vi "复材超声C扫缺陷分析评定软件.vi"() -> ()   [LabVIEW 2018]
doc: "使用该模板构建用户界面事件处理设计模式。将模板应用于对话框及其它用户界面。用户也可创建并执行VI可按照与用户界面事件相同方式处理的用户定义事件。"
uses:
  <vilib>/Utility/NIReport.llb/Report Type.ctl
  <vilib>/addons/_office/_exclsub.llb/font.ctl
  <vilib>/addons/_office/word.llb/Word Easy Table (str).vi
  <vilib>/Utility/NIReport.llb/Append Image to Report (path wrap).vi
  <vilib>/Utility/NIReport.llb/NI_report.lvclass
  <vilib>/Utility/NIReport.llb/Append Report Text (str wrap).vi
  <vilib>/vision/NI_Vision_Development_Module.lvlib
  <vilib>/Utility/NIReport.llb/NI_ReportGenerationCore.lvlib
  <vilib>/addons/_office/NI_ReportGenerationToolkit.lvlib
panel:
  out "连接的字符串 2":string
  out "临界面积百分比值":dbl
  out "临界Z值":i32
  out "true":bool
  out "标注后的图片路径":path
  out "弥散类检测结果合并":string[][](table)
  out "分层类检测结果合并":string[][](table)
  out "反射图原始路径":path
  out "穿透图原始路径":path
  out "弥散类检测结果":string[][](table)
  out "分层类检测结果":string[][](table)
  out "部位信息":string[](array[string])=["", "34.500000", "32.500000", "1121", "34", "54.955926", "分层类", "不合格", ""]
  out "连接的字符串":string
  in  "完成标注":bool caption="定量分析"
  out "框数":dbl
  in  "Operation":enum16{"overlay rectangle"}(ring)
  out "ROI左上角坐标":cluster{i32, i32}
  out "自定义字体":T1={"Desired Font (Application)"=enum."Application Font", "[User-specified Font]"={"Font Name"="", "Size"=12, "Strikeout?"=FALSE, "Italic?"=FALSE, "Underline?"=FALSE, "Outline?"=FALSE, "Shadow?"=FALSE, "Bold?"=FALSE, "Rotation Angle"=0.0}, "Horizontal Alignment"=0, "Vertical Alignment"=0} {"Horizontal Alignment" items=["Left", "Center", "Right"]; "Vertical Alignment" items=["Bottom", "Top", "Baseline"]}
  out "标注图ROI2Mask":T2(plugin-control)
  out "透射图最大灰度值":sgl
  out "反射图最大灰度值":sgl
  out "反射图灰度表":u32[](graph)
  out "透射图灰度表":u32[](graph)
  out "总面积":i32
  out "框组":T3(array[cluster])
  out "质量等级":string
  in  "导入反射图":bool caption="导入图片"
  out "灰度阈值":dbl
  in  "stop":bool caption="停止"
  in  "导入穿透图":bool caption="导入图片"
  in  "图像预处理":bool
  in  "自定义色彩":bool
  in  "缺陷标注":bool caption="定量分析"
  in  "查看标注":bool caption="辅助定性分析"
  in  "生成评定结果":bool caption="生成原始记录"
  in  "?":enum32{"穿透图", "反射图"}(tab)
  out "穿透图":T2(plugin-control)
  out "反射图":T2(plugin-control)
  out "产品规格":cluster{"产品长度（周长）（mm）":dbl, "产品宽度（母线长）（mm）":dbl}
  out "图像分辨率":T4
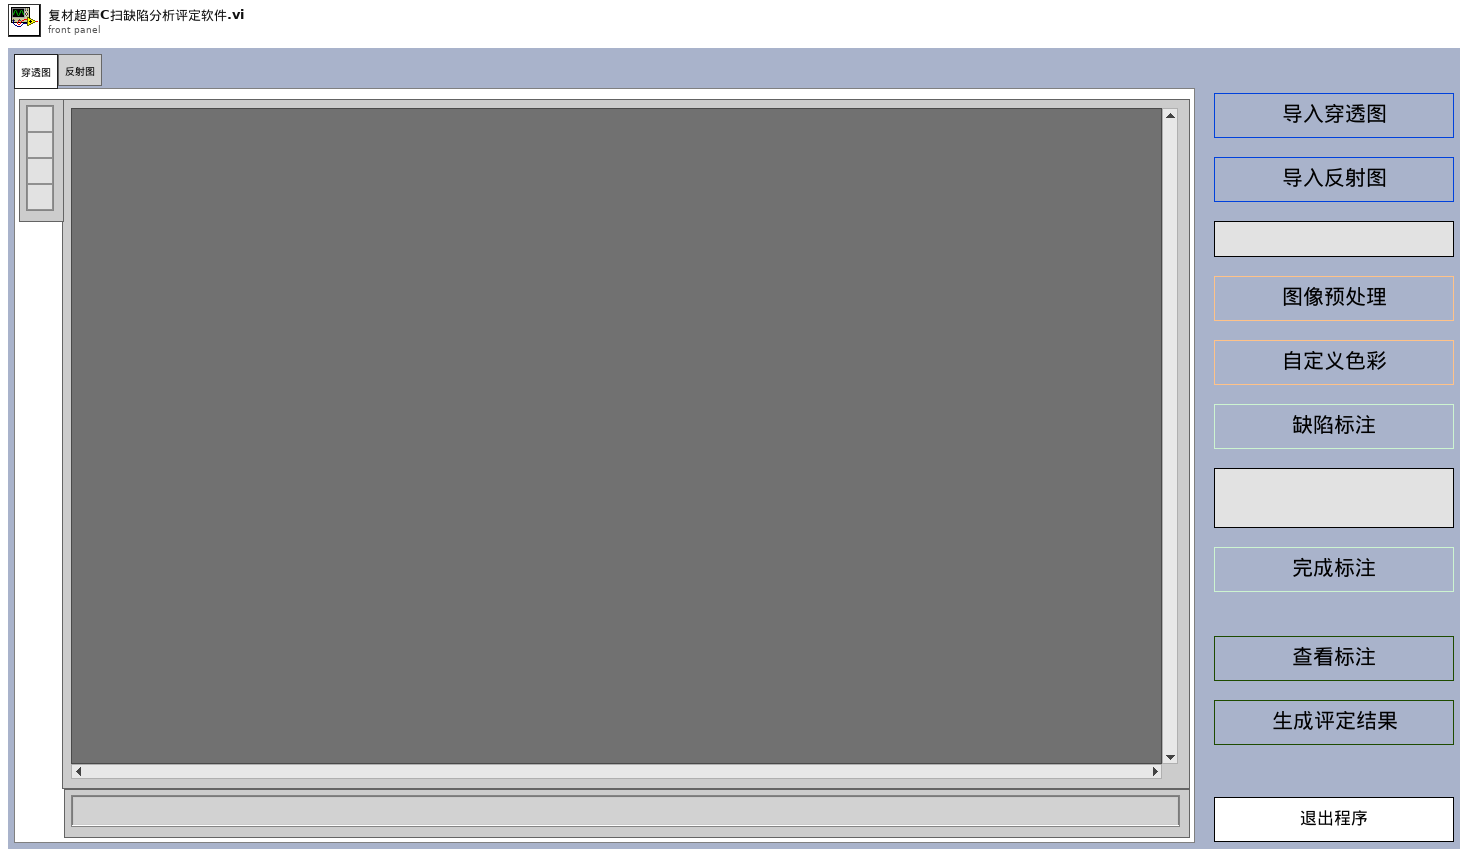
[diagram p1: front panel]
types:
  T1 = cluster{"Desired Font (Application)":enum16{"User-specified Font", "Application Font", "System Font", "Dialog Font"}, "[User-specified Font]":cluster{"Font Name":string, "Size":i16, "Strikeout?":bool, "Italic?":bool, "Underline?":bool, "Outline?":bool, "Shadow?":bool, "Bold?":bool, "Rotation Angle":dbl}, "Horizontal Alignment":i16, "Vertical Alignment":i16}
  T2 = typedef "IMAQ Image.ctl" = refnum<image>
  T3 = cluster{"Global Rectangle":i32[], "Contours":cluster{"Contour Type":u32, "ROI Type":u32, "Points":i32[]}[]}[]
  T4 = cluster{"图像X向分辨率（mm/像素）":dbl, "图像Y向分辨率（mm/像素）":dbl}
  T5 = cluster{"Zoom Tool":bool, "Selection Tool":bool, "Pan Tool":bool, "Point Tool":bool, "Line Tool":bool, "Rectangle Tool":bool, "Rotated Rectangle Tool":bool, "Polyline Tool":bool, "Polygon Tool":bool, "Freehand Tool":bool, "Closed Freehand Tool":bool, "Ellipse Tool":bool, "Annulus Tool":bool}
  T6 = enum32{"Invalid", "Standard", "Closed", "Hidden", "Minimized", "Maximized"}
  T7 = enum32{"Linear", "Log", "Exp", "Square", "Square root", "Power X", "Power 1/X"}
  T8 = enum32{"Gray", "Binary", "Gradient", "Rainbow", "Temperature"}
  T9 = cluster{"position (excel)":cluster{"row":i32, "column":i32}, "name (excel)":string, "bookmark (word)":string}
  T10 = typedef "NI_ReportGenerationToolkit.lvlib/font.ctl" = cluster{"font name":string, "font size":dbl, "bold":u16, "italic":u16, "underline":u16, "strike through":u16, "font color":u32}
  T11 = enum16{"maximized", "minimized", "normal", "no change"}
  T12 = typedef "NI_ReportGenerationCore.lvlib/Report Type.ctl" = enum16{"HTML", "Word", "Excel"}
  T13 = cluster{"position (Excel)":cluster{"row":i32, "column":i32}, "name (Excel)":string, "bookmark (Word)":string}
  T14 = typedef "Image Type" = u32
  T15 = cluster{"Red (or Hue) value":u8, "Green (or Sat) value":u8, "Blue (or Light or Val) value":u8}[]
  T16 = cluster{"histogram":u32[], "Minimal Value":sgl, "Maximal Value":sgl, "Starting Value":sgl, "Interval Width":sgl, "Mean Value":sgl, "Standard  Variation":sgl, "Area (pixels)":i32}
  T17 = cluster{"Global Rectangle":i32[], "Contours":cluster{"Contour Type":u32, "ROI Type":u32, "Points":i32[]}[]}
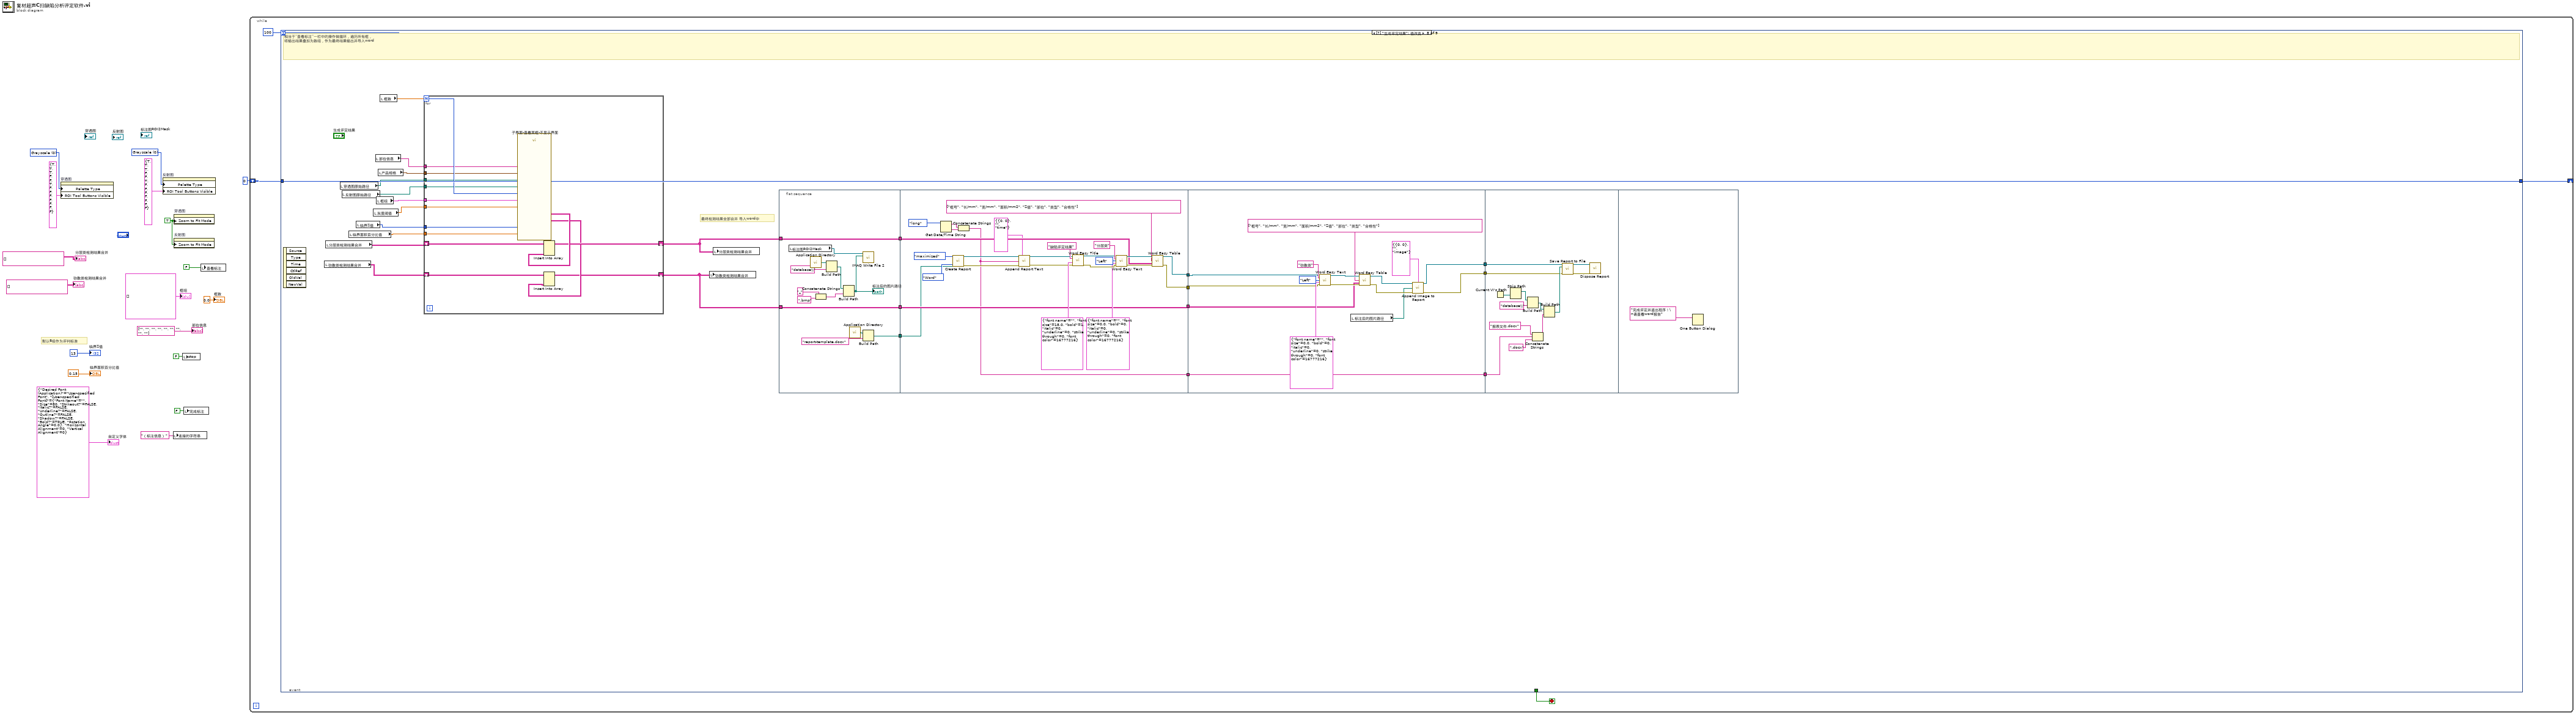
[diagram p0: block diagram]
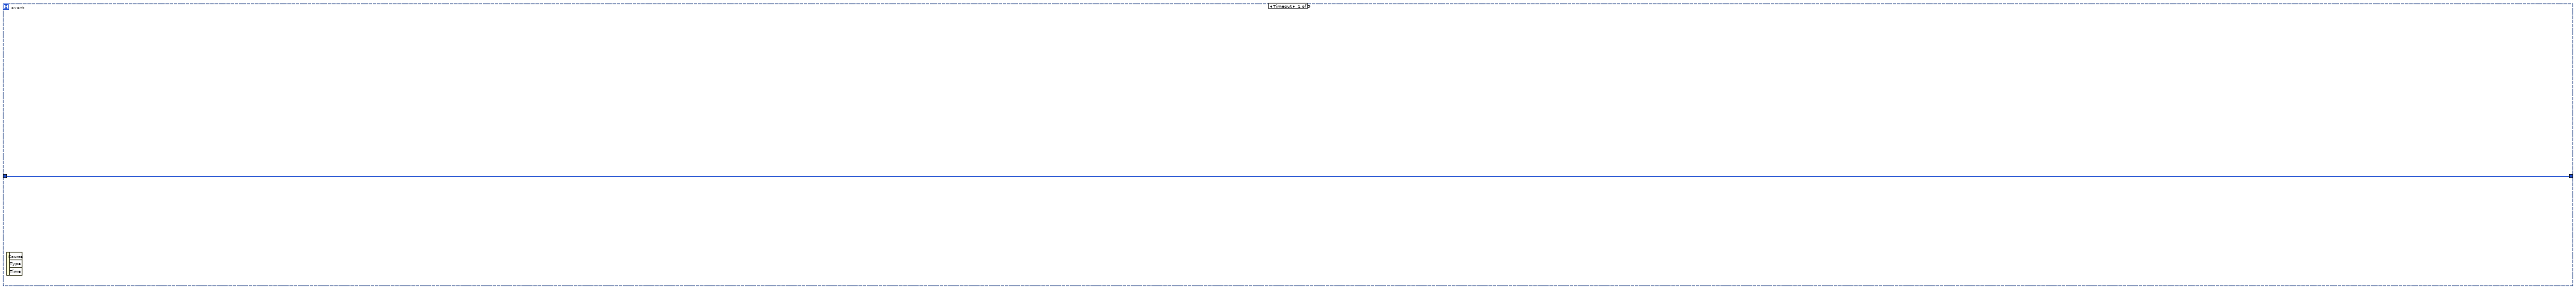
[diagram p2: hidden frame]
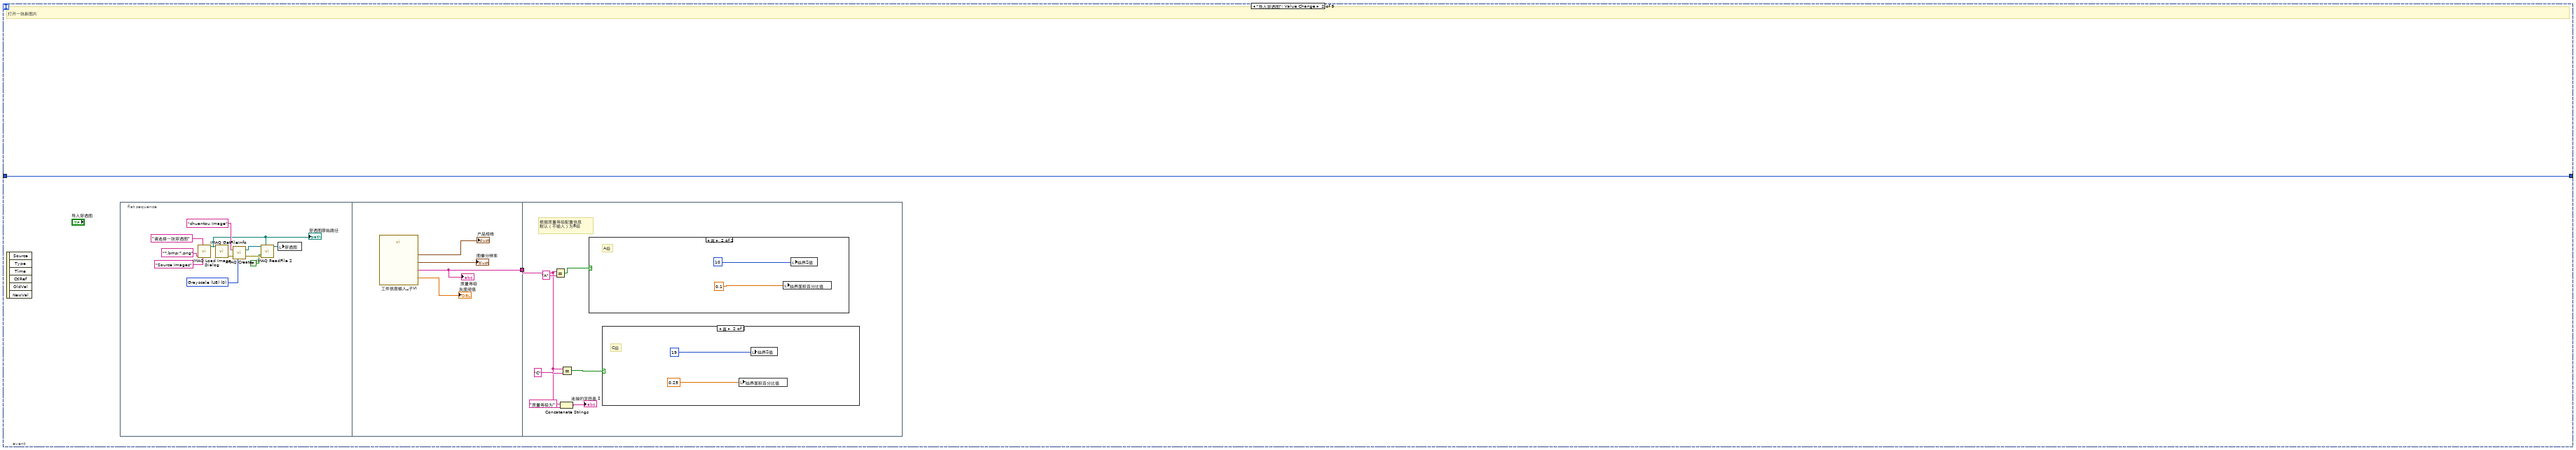
[diagram p3: hidden frame]
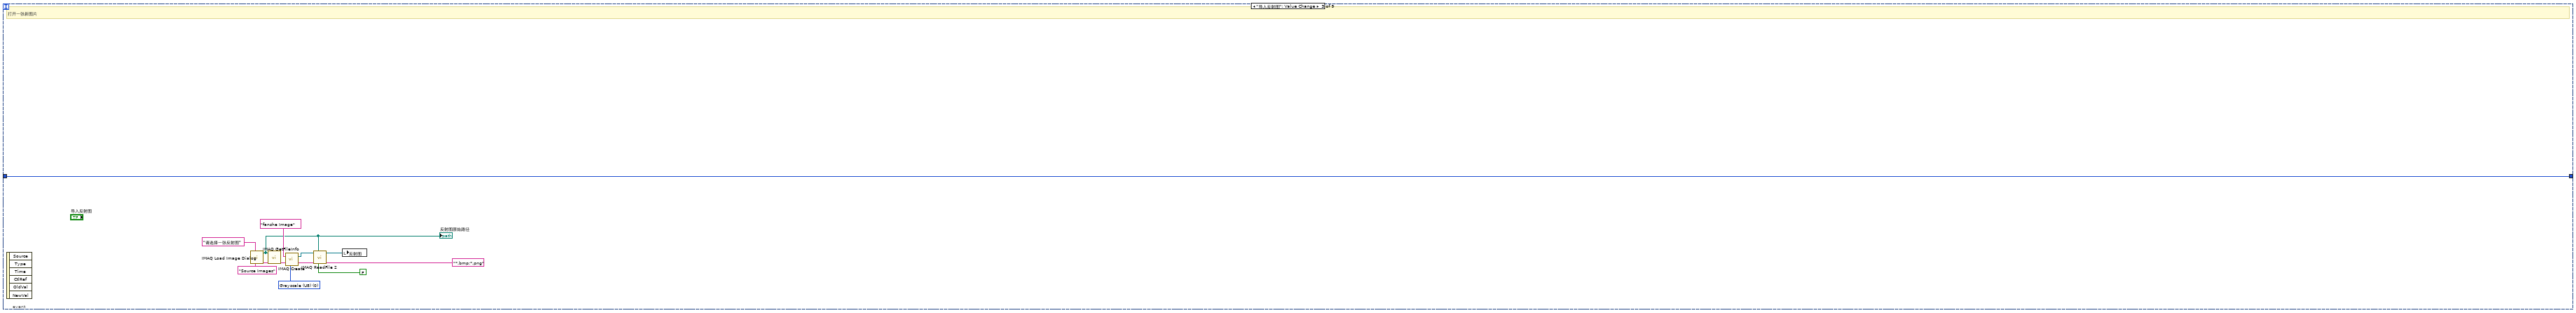
[diagram p6: hidden frame]
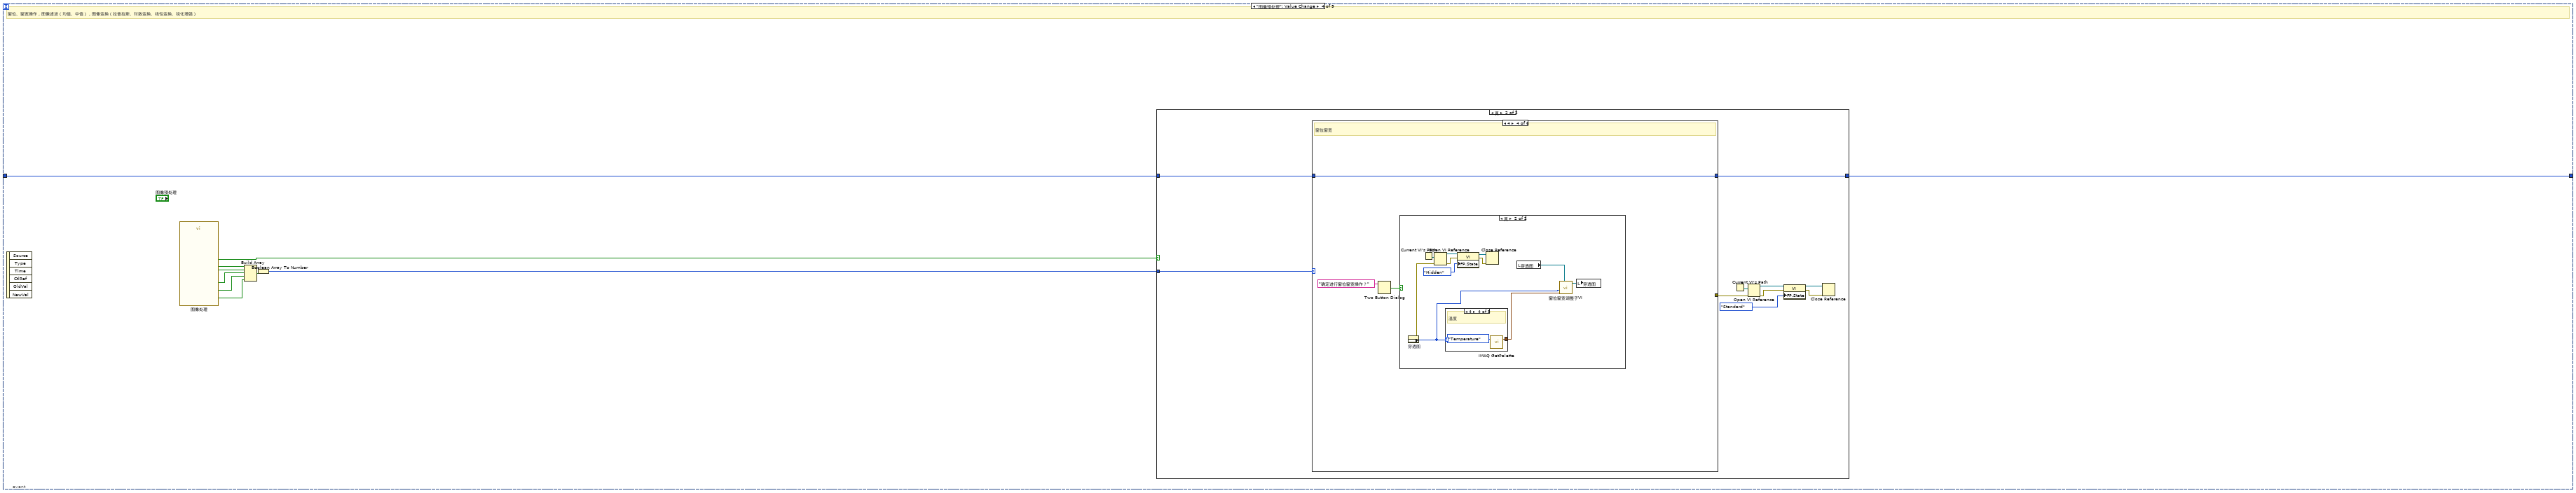
[diagram p7: hidden frame]
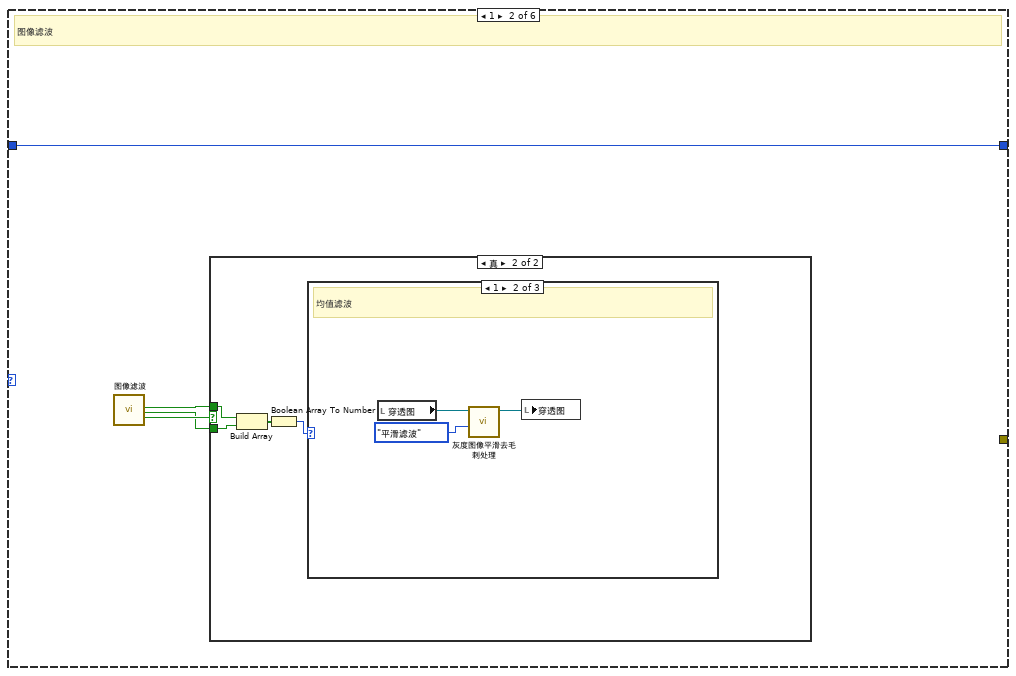
[diagram p10: hidden frame]
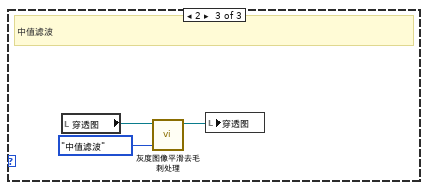
[diagram p13: hidden frame]
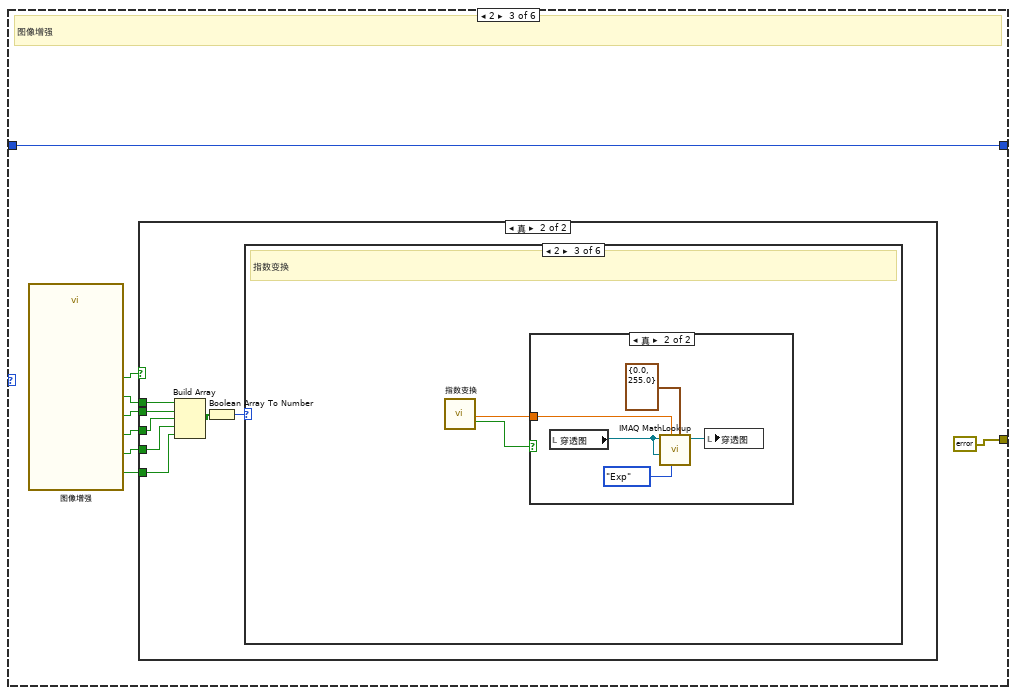
[diagram p14: hidden frame]
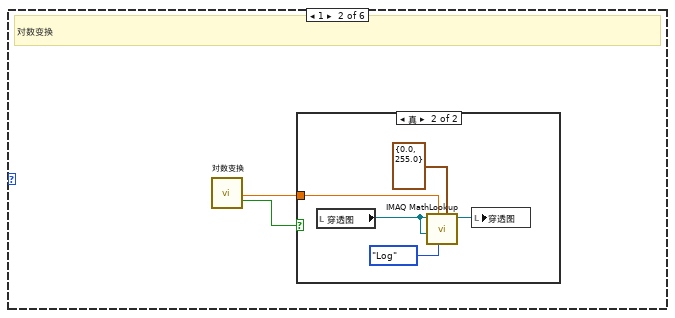
[diagram p17: hidden frame]
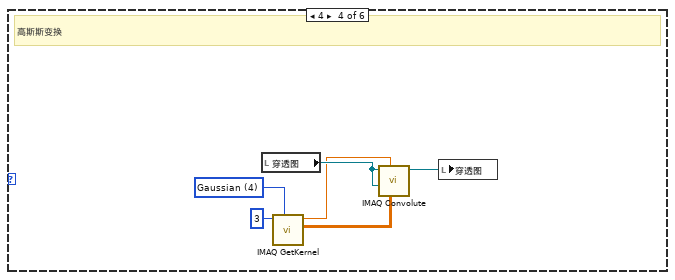
[diagram p20: hidden frame]
diagram:
  w8 = u32 0 items=["Grayscale", "Binary", "Gradient", "Rainbow", "Temperature", "User Defined", "Binary 16 Bit", "Gradient 16 Bit", "Rainbow 16 Bit", "Temperature 16 Bit", "User Defined 16 Bit"] ("Palette:Palette Type")
  w14 = TRUE ("Zoom to Fit Mode")
  w17 = u32 0 items=["Grayscale", "Binary", "Gradient", "Rainbow", "Temperature", "User Defined", "Binary 16 Bit", "Gradient 16 Bit", "Rainbow 16 Bit", "Temperature 16 Bit", "User Defined 16 Bit"] ("Palette:Palette Type")
  # "默认B级作为评判标准"
  n1 = property on="穿透图" class="ImageControl"("Palette Type"=w17, "ROI Tool Buttons Visible"=T5 {"Zoom Tool"=TRUE, "Selection Tool"=TRUE, "Pan Tool"=TRUE, "Point Tool"=FALSE, "Line Tool"=FALSE, "Rectangle Tool"=TRUE, "Rotated Rectangle Tool"=FALSE, "Polyline Tool"=FALSE, "Polygon Tool"=FALSE, "Freehand Tool"=FALSE, "Closed Freehand Tool"=FALSE, "Ellipse Tool"=FALSE, "Annulus Tool"=FALSE} ("ROI Tool Buttons Visible:All Elements")) -> ()  [unwired: 2 in, 2 out]
  n2 = property on="反射图" class="ImageControl"("Palette Type"=w8, "ROI Tool Buttons Visible"=T5 {"Zoom Tool"=TRUE, "Selection Tool"=TRUE, "Pan Tool"=TRUE, "Point Tool"=FALSE, "Line Tool"=FALSE, "Rectangle Tool"=TRUE, "Rotated Rectangle Tool"=FALSE, "Polyline Tool"=FALSE, "Polygon Tool"=FALSE, "Freehand Tool"=FALSE, "Closed Freehand Tool"=FALSE, "Ellipse Tool"=FALSE, "Annulus Tool"=FALSE} ("ROI Tool Buttons Visible:All Elements")) -> ()  [unwired: 2 in, 2 out]
  n3 = local write "连接的字符串"("（标注信息）" ("连接的字符串")) -> ()
  n4 = property on="穿透图" class="ImageControl"("Zoom to Fit Mode"=w14) -> ()  [unwired: 2 in, 2 out]
  n5 = property on="反射图" class="ImageControl"("Zoom to Fit Mode"=w14) -> ()  [unwired: 2 in, 2 out]
  n6 = local write "stop"(FALSE ("stop")) -> ()
  n7 = local write "完成标注"(FALSE ("完成标注")) -> ()
  n8 = local write "查看标注"(FALSE ("查看标注")) -> ()
  n9 = while {
    shift-right: [w19] -> _
    shift-left: 0 -> [w20]
    stop <- w22 stop-if-true
    n10 = event shown="[7] \"生成评定结果\": 值改变" {
      selector: _ -> [_ _ _ _ _ _ _ _ _]
      dyn-events: _ -> [_ _ _ _ _ _ _ _ _]
      timeout: 100 -> [_ _ _ _ _ _ _ _ _]
      tunnel: [_ _ _ _ _ _ _ _ w529] -> w22
      tunnel: w20 -> [w23 w25 w63 w65 w203 _ _ w443 _]
      tunnel: [w23 w25 w63 w64 w203 _ _ w443 0] -> w19
      event Timeout {
        n11 = event-data() -> ()  [unwired: 1 in, 3 out]
      }
      event "导入穿透图": Value Change {
        # "打开一张新图片"
        n12 = event-data() -> ()  [unwired: 1 in, 6 out]
        n13 = flat-sequence {
          tunnel: [w37] -> w24
          tunnel: w24 -> [w43]
          frame #0 {
            w28 = T14 0 items=["Grayscale (U8)", "Grayscale (I16)", "Grayscale (SGL)", "Complex (CSG)", "RGB (U32)", "HSL (U32)", "RGB (U64)", "Grayscale (U16)"] ("Image Type")
            n14 = call "IMAQ Load Image Dialog"("Pattern Label"="Source Images", "Prompt"="请选择一张穿透图" ("prompt"), "Pattern"="*.bmp;*.png") -> ("Path"=w26:path)  [unwired: 6 in, 2 out]
            "穿透图原始路径" <- w26
            n15 = call "IMAQ GetFileInfo"("File Path"=w26) -> ("error out"=w31:errorcluster)  [unwired: 4 in, 6 out]
            n16 = call "IMAQ Create"("Image Name"="chuantou Image", "Image Type"=w28, "error in (no error)"=w31) -> ("New Image"=w32:T2, "error out"=w33:errorcluster)  [unwired: 2 in]
            n17 = call "IMAQ ReadFile 2"("Use File Path Image Type"=FALSE, "File Path"=w26, "error in (no error)"=w33, "Image"=w32) -> ("Image Out"=w27:T2)  [unwired: 3 in, 4 out]
            n18 = local write "穿透图"(w27) -> ()
          }
          frame #1 {
            n19 = call "工件信息输入_子VI.vi"() -> ("质量等级"=w37:string, "灰度阈值"=→"灰度阈值":dbl, "产品规格"=→"产品规格":cluster{"产品长度（周长）（mm）":dbl, "产品宽度（母线长）（mm）":dbl}, "图像分辨率"=→"图像分辨率":T4)  [unwired: 7 in]
            "质量等级" <- w37
          }
          frame #2 {
            # "根据质量等级配置信息\n默认（不输入）为B级"
            n20 = Equal?(x=w43, y="A") -> (x = y?=w47:bool)
            n21 = Concatenate Strings("质量等级为" ("字符串"), w43) -> (→"连接的字符串 2":string)
            n22 = Equal?(x=w43, y="C") -> (x = y?=w44:bool)
            n23 = case shown="真" w47 {
              frame False {
              }
              frame True {
                # "A级"
                n24 = local write "临界面积百分比值"(0.1 ("临界面积百分比值")) -> ()
                n25 = local write "临界Z值"(10 ("临界Z值")) -> ()
              }
            }
            n26 = case shown="真" w44 {
              frame False {
              }
              frame True {
                # "C级"
                n27 = local write "临界面积百分比值"(0.25 ("临界面积百分比值")) -> ()
                n28 = local write "临界Z值"(19 ("临界Z值")) -> ()
              }
            }
          }
        }
      }
      event "导入反射图": Value Change {
        w54 = T14 0 items=["Grayscale (U8)", "Grayscale (I16)", "Grayscale (SGL)", "Complex (CSG)", "RGB (U32)", "HSL (U32)", "RGB (U64)", "Grayscale (U16)"] ("Image Type")
        # "打开一张新图片"
        n29 = event-data() -> ()  [unwired: 1 in, 6 out]
        n30 = call "IMAQ Load Image Dialog"("Pattern Label"="Source Images", "Prompt"="请选择一张反射图" ("prompt"), "Pattern"="*.bmp;*.png") -> ("Path"=w52:path)  [unwired: 6 in, 2 out]
        "反射图原始路径" <- w52
        n31 = call "IMAQ GetFileInfo"("File Path"=w52) -> ("error out"=w57:errorcluster)  [unwired: 4 in, 6 out]
        n32 = call "IMAQ Create"("Image Name"="fanshe Image", "Image Type"=w54, "error in (no error)"=w57) -> ("New Image"=w58:T2, "error out"=w59:errorcluster)  [unwired: 2 in]
        n33 = call "IMAQ ReadFile 2"("Use File Path Image Type"=FALSE, "File Path"=w52, "error in (no error)"=w59, "Image"=w58) -> ("Image Out"=w53:T2)  [unwired: 3 in, 4 out]
        n34 = local write "反射图"(w53) -> ()
      }
      event "图像预处理": Value Change {
        # "窗位、窗宽操作，图像滤波（均值、中值），图像变换（拉普拉斯、对数变换、线性变换、锐化增强）"
        n35 = event-data() -> ()  [unwired: 1 in, 6 out]
        n36 = call "图像处理"() -> ("撤销图像处理"=w66:bool, "线性灰度值测量"=w67:bool, "窗位窗宽"=w72:bool, "图像增强"=w68:bool, "图像滤波"=w73:bool, "确定"=w69:bool)  [unwired: 13 in, 1 out]
        n37 = Build Array(w73, w68, w72, w67, w66) -> (w71:bool[])
        n38 = Boolean Array To Number(Boolean array=w71) -> (number=w70:u32)
        n39 = case shown="真" w69 {
          tunnel: w70 -> [_ w84]
          tunnel: w65 -> [w74 w76]
          tunnel: [w74 w75] -> w64
          frame False {
          }
          frame True {
            n40 = case shown="4" w84 {
              tunnel: [_ _ errorcluster {"status"=FALSE, "code"=0, "source"=""} ("错误输入（无错误）") _ _ _] -> w77
              tunnel: w76 -> [w85 w86 w100 w149 w172 w194]
              tunnel: [w85 w86 w100 w149 w172 w194] -> w75
              frame 0, Default {
              }
              frame 1 {
                # "图像滤波"
                n41 = call "图像滤波"() -> ("均值滤波"=w88:bool, "中值滤波"=w87:bool, "确定"=w89:bool)  [unwired: 16 in, 1 out]
                n42 = case shown="真" w89 {
                  tunnel: w88 -> [_ w92]
                  tunnel: w87 -> [_ w91]
                  frame False {
                  }
                  frame True {
                    n43 = Build Array(w92, w91) -> (w93:bool[])
                    n44 = Boolean Array To Number(Boolean array=w93) -> (number=w90:u32)
                    n45 = case shown="1" w90 {
                      frame 0, Default {
                      }
                      frame 1 {
                        # "均值滤波"
                        n46 = local read "穿透图"() -> (w96:T2)
                        n47 = call "灰度图像平滑去毛刺处理.vi"("滤波方法选择"=enum16{"中值滤波", "平滑滤波"}."平滑滤波", "Image"=w96) -> ("Image Out"=w95:T2)  [unwired: 9 in]
                        n48 = local write "穿透图"(w95) -> ()
                      }
                      frame 2 {
                        # "中值滤波"
                        n49 = local read "穿透图"() -> (w99:T2)
                        n50 = call "灰度图像平滑去毛刺处理.vi"("滤波方法选择"=enum16{"中值滤波", "平滑滤波"}."中值滤波", "Image"=w99) -> ("Image Out"=w98:T2)  [unwired: 9 in]
                        n51 = local write "穿透图"(w98) -> ()
                      }
                    }
                  }
                }
              }
              frame 2 {
                # "图像增强"
                n52 = call "图像增强"() -> ("幂变换"=w102:bool, "阈值变换"=w103:bool, "高斯变换"=w104:bool, "指数变换"=w105:bool, "对数变换"=w106:bool, "确定"=w107:bool)  [unwired: 13 in, 1 out]
                n53 = case shown="真" w107 {
                  tunnel: w106 -> [_ w112]
                  tunnel: w105 -> [_ w111]
                  tunnel: w104 -> [_ w110]
                  tunnel: w103 -> [_ w109]
                  tunnel: w102 -> [_ w108]
                  frame False {
                  }
                  frame True {
                    n54 = Build Array(w112, w111, w110, w109, w108) -> (w114:bool[])
                    n55 = Boolean Array To Number(Boolean array=w114) -> (number=w113:u32)
                    n56 = case shown="2" w113 {
                      frame 0, Default {
                      }
                      frame 1 {
                        # "对数变换"
                        n57 = call "对数变换"() -> ("变换系数K"=w115:dbl, "确定"=w116:bool)  [unwired: 17 in, 1 out]
                        n58 = case shown="真" w116 {
                          tunnel: w115 -> [_ w117]
                          frame False {
                          }
                          frame True {
                            n59 = local read "穿透图"() -> (w121:T2)
                            n60 = call "IMAQ MathLookup"("Range"=cluster{"Minimum":sgl, "Maximum":sgl} {"Minimum"=0.0, "Maximum"=255.0}, "Operator"=T7."Log", "X Value"=w117, "Image Dst"=w121, "Image Src"=w121) -> ("Image Dst Out"=w119:T2)  [unwired: 5 in, 1 out]
                            n61 = local write "穿透图"(w119) -> ()
                          }
                        }
                      }
                      frame 2 {
                        # "指数变换"
                        n62 = call "指数变换"() -> ("变换系数K"=w122:dbl, "确定"=w123:bool)  [unwired: 17 in, 1 out]
                        n63 = case shown="真" w123 {
                          tunnel: w122 -> [_ w124]
                          frame False {
                          }
                          frame True {
                            n64 = local read "穿透图"() -> (w128:T2)
                            n65 = call "IMAQ MathLookup"("Range"=cluster{"Minimum":sgl, "Maximum":sgl} {"Minimum"=0.0, "Maximum"=255.0}, "Operator"=T7."Exp", "X Value"=w124, "Image Dst"=w128, "Image Src"=w128) -> ("Image Dst Out"=w126:T2)  [unwired: 5 in, 1 out]
                            n66 = local write "穿透图"(w126) -> ()
                          }
                        }
                      }
                      frame 4 {
                        w134 = u16 4 items=["Gradient"=1, "Laplacian"=2, "Smoothing"=3, "Gaussian"=4] ("Kernel Family")
                        # "高斯斯变换"
                        n67 = local read "穿透图"() -> (w131:T2)
                        n68 = call "IMAQ GetKernel"("Kernel Family"=w134, "Kernel Size (3,5,...)"=3) -> ("Kernel"=w132:sgl[][], "Divider"=w129:sgl)  [unwired: 6 in, 2 out]
                        n69 = call "IMAQ Convolute"("Kernel"=w132, "Divider (kernel sum)"=w129, "Image Dst"=w131, "Image Src"=w131) -> ("Image Dst Out"=w130:T2)  [unwired: 6 in, 1 out]
                        n70 = local write "穿透图"(w130) -> ()
                      }
                      frame 8 {
                        # "阈值变换"
                        n71 = call "阈值范围选择子VI.vi"() -> ("阈值范围"=w135:cluster{"Lower value":sgl, "Upper value":sgl}, "确定执行"=w136:bool)  [unwired: 10 in]
                        n72 = case shown="真" w136 {
                          tunnel: w135 -> [_ w138]
                          frame False {
                          }
                          frame True {
                            n73 = local read "穿透图"() -> (w141:T2)
                            n74 = call "IMAQ Threshold"("Replace Value"=sgl 255.0, "Keep/Replace Value (Replace)"=TRUE, "Range"=w138, "Image Dst"=w141, "Image Src"=w141) -> ("Image Dst Out"=w140:T2)  [unwired: 5 in, 1 out]
                            n75 = local write "穿透图"(w140) -> ()
                          }
                        }
                      }
                      frame 16 {
                        # "幂变换"
                        n76 = call "幂变换"() -> ("变换系数K"=w142:dbl, "确定"=w143:bool)  [unwired: 17 in, 1 out]
                        n77 = case shown="真" w143 {
                          tunnel: w142 -> [_ w144]
                          frame False {
                          }
                          frame True {
                            n78 = local read "穿透图"() -> (w148:T2)
                            n79 = call "IMAQ MathLookup"("Range"=cluster{"Minimum":sgl, "Maximum":sgl} {"Minimum"=0.0, "Maximum"=255.0}, "Operator"=T7."Power 1/X", "X Value"=w144, "Image Dst"=w148, "Image Src"=w148) -> ("Image Dst Out"=w146:T2)  [unwired: 5 in, 1 out]
                            n80 = local write "穿透图"(w146) -> ()
                          }
                        }
                      }
                    }
                  }
                }
              }
              frame 4 {
                # "窗位窗宽"
                n81 = Two Button Dialog(message="确定进行窗位窗宽操作？" ("消息")) -> (T button?=w151:bool)  [unwired: 2 in]
                n82 = case shown="真" w151 {
                  frame False {
                  }
                  frame True {
                    n83 = property on="穿透图" class="ImageControl"() -> (error out=w153:errorcluster, "Palette Type"=w160:u32)  [unwired: 2 in, 1 out]
                    n84 = Current VI's Path() -> (path=w155:path)
                    n85 = Open VI Reference(vi path=w155, error in (no error)=w153) -> (vi reference=w156:refnum<vi>, error out=w158:errorcluster)  [unwired: 4 in]
                    n86 = case shown="4" w160 {
                      tunnel: [w163 w165 w167 w169 w171] -> w161
                      frame 0, Default {
                        # "灰度"
                        n87 = call "IMAQ GetPalette"("Palette Number (gray)"=T8."Gray") -> ("Color Palette"=w163:cluster{"Red":u8, "Green":u8, "Blue":u8}[])  [unwired: 4 in, 1 out]
                      }
                      frame 2 {
                        # "梯度"
                        n88 = call "IMAQ GetPalette"("Palette Number (gray)"=T8."Gradient") -> ("Color Palette"=w165:cluster{"Red":u8, "Green":u8, "Blue":u8}[])  [unwired: 4 in, 1 out]
                      }
                      frame 3 {
                        # "彩虹"
                        n89 = call "IMAQ GetPalette"("Palette Number (gray)"=T8."Rainbow") -> ("Color Palette"=w167:cluster{"Red":u8, "Green":u8, "Blue":u8}[])  [unwired: 4 in, 1 out]
                      }
                      frame 4 {
                        # "温度"
                        n90 = call "IMAQ GetPalette"("Palette Number (gray)"=T8."Temperature") -> ("Color Palette"=w169:cluster{"Red":u8, "Green":u8, "Blue":u8}[])  [unwired: 4 in, 1 out]
                      }
                      frame 5 {
                        # "自定义"
                        n91 = property on="穿透图" class="ImageControl"() -> ("User Palette"=w171:cluster{"Red":u8, "Green":u8, "Blue":u8}[])  [unwired: 2 in, 2 out]
                      }
                    }
                    n92 = property class="VI"(reference=w156, error in=w158, "FP.State"=T6."Hidden" ("前面板窗口:状态")) -> (reference out=w157:refnum<vi>, error out=w159:errorcluster)
                    n93 = Close Reference(reference=w157, error in (no error)=w159) -> ()  [unwired: 1 out]
                    n94 = local read "穿透图"() -> (w152:T2)
                    n95 = call "窗位窗宽调整子VI.vi"("Image in"=w152, "Palette:User Palette"=w161, "Palette:Palette Type"=w160) -> ("Image out"=w162:T2)  [unwired: 8 in]
                    n96 = local write "穿透图"(w162) -> ()
                  }
                }
              }
              frame 8 {
                # "查看线灰度值曲线，用于精确测量"
                n97 = Current VI's Path() -> (path=w179:path)
                n98 = Open VI Reference(vi path=w179) -> (vi reference=w178:refnum<vi>, error out=w176:errorcluster)  [unwired: 5 in]
                n99 = property class="VI"(reference=w178, error in=w176, "FP.State"=T6."Hidden" ("前面板窗口:状态")) -> (reference out=w177:refnum<vi>, error out=w175:errorcluster)
                n100 = Close Reference(reference=w177, error in (no error)=w175) -> (error out=w173:errorcluster)
                n101 = case shown="无错误" w173 {
                  frame No Error {
                    n102 = property on="穿透图" class="ImageControl"() -> ("Palette Type"=w181:u32)  [unwired: 2 in, 2 out]
                    n103 = case shown="2" w181 {
                      tunnel: [w184 w186 w188 w190 w192] -> w180
                      frame 0, Default {
                        # "灰度"
                        n104 = call "IMAQ GetPalette"("Palette Number (gray)"=T8."Gray") -> ("Color Palette"=w184:cluster{"Red":u8, "Green":u8, "Blue":u8}[])  [unwired: 4 in, 1 out]
                      }
                      frame 2 {
                        # "梯度"
                        n105 = call "IMAQ GetPalette"("Palette Number (gray)"=T8."Gradient") -> ("Color Palette"=w186:cluster{"Red":u8, "Green":u8, "Blue":u8}[])  [unwired: 4 in, 1 out]
                      }
                      frame 3 {
                        # "彩虹"
                        n106 = call "IMAQ GetPalette"("Palette Number (gray)"=T8."Rainbow") -> ("Color Palette"=w188:cluster{"Red":u8, "Green":u8, "Blue":u8}[])  [unwired: 4 in, 1 out]
                      }
                      frame 4 {
                        # "温度"
                        n107 = call "IMAQ GetPalette"("Palette Number (gray)"=T8."Temperature") -> ("Color Palette"=w190:cluster{"Red":u8, "Green":u8, "Blue":u8}[])  [unwired: 4 in, 1 out]
                      }
                      frame 5 {
                        # "自定义"
                        n108 = property on="穿透图" class="ImageControl"() -> ("User Palette"=w192:cluster{"Red":u8, "Green":u8, "Blue":u8}[])  [unwired: 2 in, 2 out]
                      }
                    }
                    n109 = local read "穿透图"() -> (w183:T2)
                    n110 = local read "图像分辨率"() -> (w182:T4)
                    n111 = call "线性灰度值曲线查看子VI.vi"("Palette:User Palette"=w180, "图像分辨率"=w182, "Image"=w183) -> ()  [unwired: 9 in]
                  }
                  frame Error {
                  }
                }
              }
              frame 16 {
                # "撤销图像处理，恢复原图"
                n112 = call "IMAQ Create"("Image Name"="P1") -> ("New Image"=w193:T2)  [unwired: 4 in, 1 out]
                n113 = local write "穿透图"(w193) -> ()
              }
            }
            n114 = Current VI's Path() -> (path=w83:path)
            n115 = Open VI Reference(vi path=w83, error in (no error)=w77) -> (vi reference=w82:refnum<vi>, error out=w79:errorcluster)  [unwired: 4 in]
            n116 = property class="VI"(reference=w82, error in=w79, "FP.State"=T6."Standard" ("前面板窗口:状态")) -> (reference out=w80:refnum<vi>, error out=w78:errorcluster)
            n117 = Close Reference(reference=w80, error in (no error)=w78) -> ()  [unwired: 1 out]
          }
        }
      }
      event "自定义色彩": Value Change {
        # "色彩、色阶自定义"
        n118 = event-data() -> ()  [unwired: 1 in, 6 out]
        n119 = call "调色板"() -> ("自定义显示"=w197:bool, "温度显示"=w198:bool, "彩虹显示"=w199:bool, "梯度显示"=w200:bool, "灰度显示"=w201:bool, "确定"=w202:bool)  [unwired: 13 in, 1 out]
        n120 = Build Array(w201, w200, w199, w198, w197) -> (w196:bool[])
        n121 = case shown="假" w202 {
          tunnel: w196 -> [_ w206]
          frame False {
          }
          frame True {
            n122 = Boolean Array To Number(Boolean array=w206) -> (number=w205:u32)
            n123 = case shown="16" w205 {
              tunnel: [w207 w208 w209 w210 w211 w213] -> w204
              frame 0, Default {
                w207 = u32 0 items=["Grayscale", "Binary", "Gradient", "Rainbow", "Temperature", "User Defined", "Binary 16 Bit", "Gradient 16 Bit", "Rainbow 16 Bit", "Temperature 16 Bit", "User Defined 16 Bit"] ("Palette:Palette Type")
              }
              frame 1 {
                w208 = u32 0 items=["Grayscale", "Binary", "Gradient", "Rainbow", "Temperature", "User Defined", "Binary 16 Bit", "Gradient 16 Bit", "Rainbow 16 Bit", "Temperature 16 Bit", "User Defined 16 Bit"] ("Palette:Palette Type")
                # "灰度"
              }
              frame 2 {
                w209 = u32 2 items=["Grayscale", "Binary", "Gradient", "Rainbow", "Temperature", "User Defined", "Binary 16 Bit", "Gradient 16 Bit", "Rainbow 16 Bit", "Temperature 16 Bit", "User Defined 16 Bit"] ("Palette:Palette Type")
                # "梯度"
              }
              frame 4 {
                w210 = u32 3 items=["Grayscale", "Binary", "Gradient", "Rainbow", "Temperature", "User Defined", "Binary 16 Bit", "Gradient 16 Bit", "Rainbow 16 Bit", "Temperature 16 Bit", "User Defined 16 Bit"] ("Palette:Palette Type")
                # "彩虹"
              }
              frame 8 {
                w211 = u32 4 items=["Grayscale", "Binary", "Gradient", "Rainbow", "Temperature", "User Defined", "Binary 16 Bit", "Gradient 16 Bit", "Rainbow 16 Bit", "Temperature 16 Bit", "User Defined 16 Bit"] ("Palette:Palette Type")
                # "温度"
              }
              frame 16 {
                w213 = u32 5 items=["Grayscale", "Binary", "Gradient", "Rainbow", "Temperature", "User Defined", "Binary 16 Bit", "Gradient 16 Bit", "Rainbow 16 Bit", "Temperature 16 Bit", "User Defined 16 Bit"] ("Palette:Palette Type")
                # "自定义"
                n124 = call "自定义成像色谱20200214.vi"() -> ("Color palette"=w212:T15)  [unwired: 8 in, 1 out]
                n125 = property on="穿透图" class="ImageControl"("User Palette"=w212) -> ()  [unwired: 2 in, 2 out]
              }
            }
            n126 = property on="穿透图" class="ImageControl"("Palette Type"=w204) -> ()  [unwired: 2 in, 2 out]
          }
        }
      }
      event "缺陷标注": Value Change {
        # "手动画框ROI，提取框组（坐标）、框数等信息 \n并同时也要进行阈值分割、缺陷特征提取 \n有关数据将存储并用于后续的生成评定结果"
        n127 = event-data() -> ()  [unwired: 1 in, 6 out]
        n128 = One Button Dialog(message="开始标注！\n全部标注完成后，\n请点击“完成标注”按钮" ("消息")) -> ()  [unwired: 1 in, 1 out]
        n129 = while {
          shift-right: [w238] -> _
          shift-left: _ -> [w237]
          tunnel: [w223] -> _
          tunnel: [w222] -> _
          stop <- w219 stop-if-true
          (unwired) "_" ("名称或相对路径")
          (unwired) ".docx" ("名称或相对路径")
          w221 = i32[] [2] items=["No Event"=0, "Click Event"=1, "Draw Event"=2, "Size Event"=4, "Scroll Event"=5, "Double Click Event"=8] ("Which Events")
          # "循环的方式给输入图像手动画框"
          n130 = local read "穿透图"() -> (w227:T2)
          n131 = local read "反射图"() -> (w228:T2)
          n132 = invoke on="穿透图" class="ImageControl" method="Get Last Event"("Which Events"=w221) -> ("Type"=w220:i32)  [unwired: 7 in, 7 out]
          n133 = call "IMAQ Histogram"("Number of Classes"=256, "Interval Range"=cluster{"Minimum":sgl, "Maximum":sgl} {"Minimum"=0.0, "Maximum"=255.0}, "Image"=w228) -> ("Histogram Report"=w230:T16)  [unwired: 7 in, 1 out]
          n134 = call "IMAQ Histogram"("Number of Classes"=256, "Interval Range"=cluster{"Minimum":sgl, "Maximum":sgl} {"Minimum"=0.0, "Maximum"=255.0}, "Image"=w227) -> ("Histogram Report"=w232:T16)  [unwired: 7 in, 1 out]
          n135 = Unbundle(w230) -> ("histogram"=→"反射图灰度表":u32[], "Maximal Value"=→"反射图最大灰度值":sgl)  [unwired: 6 out]
          n136 = Unbundle(w232) -> ("histogram"=→"透射图灰度表":u32[], "Maximal Value"=→"透射图最大灰度值":sgl, "Area (pixels)"=→"总面积":i32)  [unwired: 5 out]
          n137 = Not Equal To 0?(x=w220) -> (x != 0?=w239:bool)
          n138 = case shown="真" w239 {
            tunnel: w227 -> [w283 w291]
            tunnel: [w283 w290] -> w223
            tunnel: "Operation" -> [_ w289]
            tunnel: [w281 w284] -> w238
            tunnel: w237 -> [w281 w288]
            tunnel: w228 -> [w280 w287]
            tunnel: [w280 w286] -> w222
            frame False {
              n139 = Wait (ms)(milliseconds to wait=u32 50) -> ()  [unwired: 1 out]
            }
            frame True {
              n140 = property on="穿透图" class="ImageControl"() -> ("ROI"=w285:T17)  [unwired: 2 in, 2 out]
              n141 = case shown="\"overlay rectangle\"" w289 {
                tunnel: w291 -> [w310]
                tunnel: w285 -> [w308]
                tunnel: [w309] -> w290
                tunnel: w288 -> [w307]
                tunnel: w287 -> [w306]
                tunnel: [w305] -> w286
                tunnel: [w304] -> w284
                frame "overlay rectangle" {
                  n142 = flat-sequence {
                    tunnel: w310 -> [w312]
                    tunnel: [w312] -> w303
                    tunnel: w308 -> [w315]
                    tunnel: [w315] -> w302
                    tunnel: w307 -> [w314]
                    tunnel: w306 -> [w311]
                    tunnel: [w311] -> w301
                    tunnel: [w313] -> w300
                    tunnel: w303 -> [w324]
                    tunnel: w302 -> [w323]
                    tunnel: w301 -> [w329]
                    tunnel: w300 -> [w321]
                    tunnel: [w330] -> w299
                    tunnel: [w328] -> w298
                    tunnel: [w321] -> w297
                    tunnel: [w318] -> w296
                    tunnel: [w316] -> w292
                    tunnel: w299 -> [w354]
                    tunnel: w298 -> [w353]
                    tunnel: w297 -> [w352]
                    tunnel: w296 -> [w343]
                    tunnel: [w354] -> w295
                    tunnel: [w353] -> w294
                    tunnel: [w352] -> w293
                    tunnel: w292 -> [w339]
                    tunnel: [w361] -> w304
                    tunnel: [w362] -> w305
                    tunnel: [w363] -> w309
                    tunnel: w295 -> [w363]
                    tunnel: w294 -> [w362]
                    tunnel: w293 -> [w361]
                    frame #0 {
                      # "将当前ROI数据存入框组内"
                      n143 = Build Array (concatenate)(w314, w315) -> (w313:T3)
                      n144 = local write "框组"(w313) -> ()
                    }
                    frame #1 {
                      w326 = u32[] [0] ("Colors (Green)")
                      w322 = u32 16711776 ("Text Color (black)")
                      # "在反射图上对应位置画框"
                      # "在穿透图上画框"
                      # "图层名Group与“框&图层计数”变量同名，\neg：1号框对应group1"
                      # "overlay text在ROI的左上角添加计数显示"
                      # "overlay ROI代表用户手画绿色框的图层添加"
                      n145 = Unbundle(w323) -> ("Global Rectangle"=w336:i32[])  [unwired: 1 out]
                      n146 = local read "框组"() -> (w333:T3)
                      n147 = Index Array(array=w336, index=0 ("索引")) -> (element=w335:i32)
                      n148 = Index Array(array=w336, index=1 ("索引")) -> (element=w334:i32)
                      n149 = Array Size(array=w333) -> (size(s)=w316:i32)
                      n150 = Bundle(w335, w334) -> (w325:cluster{i32, i32})  [unwired: 1 in]
                      "ROI左上角坐标" <- w325
                      n151 = Number To Decimal String(number=w316) -> (decimal integer string=w317:string)  [unwired: 1 in]
                      n152 = Concatenate Strings(w317, "#" ("字符串")) -> (w318:string)
                      n153 = call "IMAQ Overlay ROI"("Colors (Green)"=w326, "Group"=w318, "ROI Descriptor"=w323, "Image"=w324) -> ("Image Out"=w337:T2)  [unwired: 6 in, 1 out]
                      n154 = call "IMAQ Overlay ROI"("Colors (Green)"=w326, "Group"=w318, "ROI Descriptor"=w323, "Image"=w329) -> ("Image Out"=w327:T2)  [unwired: 6 in, 1 out]
                      n155 = local write "框数"(w316) -> ()
                      n156 = local read "自定义字体"() -> (w320:T1)
                      n157 = call "IMAQ Overlay Text"("Group"=w318, "Text Color (black)"=w322, "Font, Size & Style"=w320, "String"=w318, "Origin"=w325, "Image"=w337) -> ("Image Out"=w330:T2)  [unwired: 4 in, 1 out]
                      n158 = call "IMAQ Overlay Text"("Group"=w318, "Text Color (black)"=w322, "Font, Size & Style"=w320, "String"=w318, "Origin"=w325, "Image"=w327) -> ("Image Out"=w328:T2)  [unwired: 4 in, 1 out]
                    }
                    frame #2 {
                      # "存放部位信息的1D数组，后续生成报告使用"
                      # "0：位于蒙皮部位\n1：位于筋条部位"
                      n159 = call "缺陷部位标注"() -> ("位于筋条处"=w348:bool, "位于蒙皮处"=w347:bool)  [unwired: 16 in, 2 out]
                      n160 = Decrement(x=w339) -> (x-1=w338:i32)
                      n161 = local read "部位信息"() -> (w342:string[])
                      n162 = Build Array(w347, w348) -> (w349:bool[])
                      n163 = Boolean Array To Number(Boolean array=w349) -> (number=w350:u32)
                      n164 = case shown="1, 默认" w350 {
                        tunnel: ["蒙皮处" ("t") "筋条处" ("t")] -> w341
                        frame 1, Default {
                        }
                        frame 2 {
                        }
                      }
                      n165 = Concatenate Strings("框号为" ("字符串"), w343, "\n", "类别为" ("字符串"), w341) -> (→"连接的字符串":string)
                      n166 = Insert Into Array(array=w342, index=w338, new element=w341) -> (w340:string[])
                      n167 = local write "部位信息"(w340) -> ()
                    }
                    frame #3 {
                      n168 = Two Button Dialog(message="是否需要删除标注" ("消息"), 1:"是" ("F按钮名称（“取消”）"), 2:"否" ("T按钮名称（“确定”）")) -> (T button?=w359:bool)
                      n169 = case shown="假" w359 {
                        frame False {
                          n170 = call "用户输入"() -> ("框号"=w364:dbl, "确定"=w365:bool)  [unwired: 17 in, 1 out]
                          n171 = case shown="真" w365 {
                            tunnel: w364 -> [_ w366]
                            frame False {
                              # "用户取消操作"
                            }
                            frame True {
                              n172 = stacked-sequence {
                                tunnel: w366 -> [_ w374 _]
                                frame #0 {
                                # "1. 删除所有框"
                                n173 = local read "反射图"() -> (w368:T2)
                                n174 = local read "穿透图"() -> (w367:T2)
                                n175 = call "IMAQ Clear Overlay"("Image"=w368) -> ()  [unwired: 9 in, 2 out]
                                n176 = call "IMAQ Clear Overlay"("Image"=w367) -> ()  [unwired: 9 in, 2 out]
                                }
                                frame #1 {
                                # "2. 删除框组中指定元素"
                                n177 = local read "部位信息"() -> (w371:string[])
                                n178 = local read "框组"() -> (w373:T3)
                                n179 = Decrement(x=w374) -> (x-1=w370:dbl)
                                n180 = Delete From Array(array=w371, index=w370) -> (array with subset deleted=w369:string[])  [unwired: 1 in, 1 out]
                                n181 = Delete From Array(array=w373, index=w370) -> (array with subset deleted=w372:T3)  [unwired: 1 in, 1 out]
                                n182 = local write "框组"(w372) -> ()
                                n183 = local write "部位信息"(w369) -> ()
                                }
                                frame #2 {
                                # "3. 重画所有框"
                                n184 = while {
                                i -> [w389]
                                stop <- w378 stop-if-true
                                n185 = local read "框组"() -> (w382:T3)
                                n186 = local read "穿透图"() -> (w388:T2)
                                n187 = local read "反射图"() -> (w383:T2)
                                n188 = Array Size(array=w382) -> (size(s)=w385:i32)
                                n189 = Index Array(array=w382, index=w389) -> (element=w377:T17)
                                n190 = Increment(x=w389) -> (x+1=w398:i32)
                                n191 = Unbundle(w377) -> ("Global Rectangle"=w386:i32[])  [unwired: 1 out]
                                n192 = call "IMAQ Overlay ROI"("ROI Descriptor"=w377, "Image"=w388) -> ("Image Out"=w396:T2)  [unwired: 8 in, 1 out]
                                n193 = call "IMAQ Overlay ROI"("ROI Descriptor"=w377, "Image"=w383) -> ("Image Out"=w391:T2)  [unwired: 8 in, 1 out]
                                n194 = Greater Or Equal?(x=w398, y=w385) -> (x >= y?=w378:bool)
                                n195 = local read "自定义字体"() -> (w376:T1)
                                n196 = Index Array(array=w386, index=1 ("索引")) -> (element=w394:i32)
                                n197 = Index Array(array=w386, index=0 ("索引")) -> (element=w393:i32)
                                n198 = Bundle(w393, w394) -> (w380:cluster{i32, i32})  [unwired: 1 in]
                                n199 = Number To Decimal String(number=w398) -> (decimal integer string=w379:string)  [unwired: 1 in]
                                n200 = Concatenate Strings(w379, "#" ("字符串")) -> (w375:string)
                                n201 = call "IMAQ Overlay Text"("Text Color (black)"=u32 16711680, "Font, Size & Style"=w376, "String"=w375, "Origin"=w380, "Image"=w391) -> ("Image Out"=w384:T2)  [unwired: 5 in, 1 out]
                                n202 = call "IMAQ Overlay Text"("Text Color (black)"=u32 16711680, "Font, Size & Style"=w376, "String"=w375, "Origin"=w380, "Image"=w396) -> ("Image Out"=w387:T2)  [unwired: 5 in, 1 out]
                                n203 = local write "反射图"(w384) -> ()
                                n204 = local write "穿透图"(w387) -> ()
                                n205 = local write "框数"(w385) -> ()
                                }
                                }
                              }
                            }
                          }
                        }
                        frame True {
                        }
                      }
                    }
                  }
                }
              }
            }
          }
          n206 = disable-structure shown="禁用" {
            frame Disabled {
              n207 = local read "查看标注"() -> (w242:bool)
              n208 = case shown="真" w242 {
                selector: w242 -> [w243 _]
                tunnel: [w243 w244] -> w241
                frame False {
                }
                frame True {
                  n209 = One Button Dialog(message="请先点击“完成标注”按钮！" ("消息")) -> (true=w244:bool)  [unwired: 1 in]
                }
              }
              "true" <- w241
            }
            frame Enabled {
            }
          }
          n210 = case shown="真" "完成标注" {
            tunnel: [FALSE ("T button?") w248] -> w217
            frame False {
            }
            frame True {
              n211 = Two Button Dialog(message="请确认是否完成标注" ("消息")) -> (T button?=w248:bool)  [unwired: 2 in]
            }
          }
          n212 = case shown="真" w217 {
            tunnel: [FALSE w250] -> w216
            frame False {
            }
            frame True {
              n213 = while {
                tunnel: [w255] -> w250
                i -> [w261]
                stop <- w255 stop-if-true
                w266 = 2 items=["White", "Black", "Inverted", "Black on White", "White on Black"] ("Color")
                w270 = u16 2 items=["Frame", "Paint", "Invert Frame", "Invert Paint"] ("Draw Mode")
                w263 = u16 1 items=["Line", "Rectangle", "Oval"] ("Shape to draw")
                # "生成绘制了ROI的图像\n可以用于后续的图片导出保存"
                n214 = local read "框组"() -> (w260:T3)
                n215 = local read "穿透图"() -> (w257:T2)
                n216 = local read "标注图ROI2Mask"() -> (w256:T2)
                n217 = Array Size(array=w260) -> (size(s)=w278:i32)
                n218 = Index Array(array=w260, index=w261) -> (element=w259:T17)
                n219 = Unbundle(w259) -> ("Global Rectangle"=w258:i32[])  [unwired: 1 out]
                n220 = Increment(x=w261) -> (x+1=w279:i32)
                n221 = Greater Or Equal?(x=w279, y=w278) -> (x >= y?=w255:bool)
                n222 = Index Array(array=w258, index=0 ("索引")) -> (element=w268:i32)
                n223 = Index Array(array=w258, index=2 ("索引")) -> (element=w273:i32)
                n224 = Index Array(array=w258, index=1 ("索引")) -> (element=w267:i32)
                n225 = Index Array(array=w258, index=3 ("索引")) -> (element=w272:i32)
                n226 = Number To Decimal String(number=w279) -> (decimal integer string=w264:string)  [unwired: 1 in]
                n227 = Build Array(w268, w267, w273, w272) -> (w251:i32[])
                n228 = call "IMAQ Draw"("Draw Mode"=w270, "Shape to draw"=w263, "Pixel Color"=sgl 0.0, "Coordinates"=w251, "Image Dst"=w256, "Image Src"=w257) -> ("Image Dst Out"=w269:T2)  [unwired: 4 in, 1 out]
                n229 = Concatenate Strings(w264, "#" ("字符串")) -> (w262:string)
                n230 = local read "自定义字体"() -> (w253:T1)
                n231 = Build Array(w268, w267) -> (w254:i32[])
                n232 = call "IMAQ Draw Text"("String"=w262, "Insertion Point"=w254, "Color"=w266, "Font, Size & Style"=w253, "Image Dst"=w256, "Image Src"=w269) -> ("Image Dst Out"=w252:T2)  [unwired: 2 in, 3 out]
                n233 = local write "标注图ROI2Mask"(w252) -> ()
              }
            }
          }
          n234 = local write "穿透图"(w223) -> ()
          n235 = local write "反射图"(w222) -> ()
          n236 = local read "stop"() -> (w218:bool)
          n237 = Or(x=w218, y=w216) -> (x .or. y?=w219:bool)
          n238 = call <vilib>:"Application Directory.vi"() -> ()  [unwired: 1 out]
        }
      }
      event "查看标注": Value Change {
        # "查看指定框的详细信息，包括灰度和面积阈值分割后的结果，提取到的长宽面积等信息"
        n239 = event-data() -> ()  [unwired: 1 in, 6 out]
        n240 = local read "部位信息"() -> (w404:string[])
        n241 = local read "反射图原始路径"() -> (w402:path)
        n242 = local read "穿透图原始路径"() -> (w403:path)
        n243 = local read "产品规格"() -> (w405:cluster{"产品长度（周长）（mm）":dbl, "产品宽度（母线长）（mm）":dbl})
        n244 = local read "临界面积百分比值"() -> (w399:dbl)
        n245 = local read "灰度阈值"() -> (w406:dbl)
        n246 = local read "框组"() -> (w401:T3)
        n247 = call "输入选择框号"() -> ("框号"=w408:dbl, "确定"=w407:bool)  [unwired: 17 in, 1 out]
        n248 = local read "临界Z值"() -> (w400:i32)
        n249 = case shown="真" w407 {
          tunnel: w408 -> [_ w419]
          tunnel: w406 -> [_ w418]
          tunnel: w405 -> [_ w417]
          tunnel: w404 -> [_ w414]
          tunnel: w403 -> [_ w413]
          tunnel: w402 -> [_ w412]
          tunnel: w401 -> [_ w411]
          tunnel: w400 -> [_ w410]
          tunnel: w399 -> [_ w409]
          frame False {
            # "用户取消操作"
          }
          frame True {
            n250 = call "子界面-查看某框.vi"("框号"=w419, "框组"=w411, "临界Z值"=w410, "反射图原始路径"=w412, "临界面积百分比值"=w409, "预先配置的灰度阈值"=w418, "穿透图原始路径"=w413, "部位信息"=w414, "产品规格"=w417) -> ("弥散类检测结果"=→"弥散类检测结果":string[][], "分层类检测结果"=→"分层类检测结果":string[][])  [unwired: 9 in]
          }
        }
      }
      event "生成评定结果": Value Change {
        # "最终检测结果全部合并 导入word中"
        # "相当于“查看标注”一栏中的操作做循环，遍历所有框，\n将输出结果叠加为数组，作为最终结果输出并导入word"
        n251 = event-data() -> ()  [unwired: 1 in, 6 out]
        n252 = local read "弥散类检测结果合并"() -> (w434:string[][])
        n253 = local read "分层类检测结果合并"() -> (w435:string[][])
        n254 = local read "穿透图原始路径"() -> (w437:path)
        n255 = local read "反射图原始路径"() -> (w436:path)
        n256 = local read "临界面积百分比值"() -> (w420:dbl)
        n257 = local read "临界Z值"() -> (w421:i32)
        n258 = local read "灰度阈值"() -> (w440:dbl)
        n259 = local read "部位信息"() -> (w439:string[])
        n260 = local read "框组"() -> (w441:T3)
        n261 = local read "产品规格"() -> (w438:cluster{"产品长度（周长）（mm）":dbl, "产品宽度（母线长）（mm）":dbl})
        n262 = local read "框数"() -> (w442:dbl)
        n263 = for {
          N: w442 -> [w526]
          tunnel: w441 -> [w527]
          tunnel: w440 -> [w525]
          tunnel: w439 -> [w524]
          tunnel: w438 -> [w523]
          tunnel: w437 -> [w522]
          tunnel: w436 -> [w521]
          shift-right: [w517] -> w433
          shift-left: w435 -> [w520]
          shift-right: [w515] -> w431
          shift-left: w434 -> [w519]
          tunnel: w421 -> [w514]
          tunnel: w420 -> [w513]
          n264 = call "子界面-查看某框-不显示界面.vi"("框号"=w526, "框组"=w527, "临界Z值"=w514, "反射图原始路径"=w521, "临界面积百分比值"=w513, "预先配置的灰度阈值"=w525, "穿透图原始路径"=w522, "部位信息"=w524, "产品规格"=w523) -> ("弥散类检测结果"=w516:string[][], "分层类检测结果"=w518:string[][])  [unwired: 9 in]
          n265 = Insert Into Array(array=w520, new element=w518) -> (w517:string[][])  [unwired: 2 in]
          n266 = Insert Into Array(array=w519, new element=w516) -> (w515:string[][])  [unwired: 2 in]
        }
        n267 = local write "弥散类检测结果合并"(w431) -> ()
        n268 = local write "分层类检测结果合并"(w433) -> ()
        n269 = flat-sequence {
          tunnel: w431 -> [w455]
          tunnel: w433 -> [w456]
          tunnel: [w456] -> w428
          tunnel: [w455] -> w427
          tunnel: [w445] -> w426
          tunnel: [w469] -> w432
          tunnel: [w468] -> w430
          tunnel: [w467] -> w429
          tunnel: w428 -> [w470]
          tunnel: w427 -> [w469]
          tunnel: w426 -> [w466]
          tunnel: [w459] -> w423
          tunnel: w432 -> [w492]
          tunnel: w430 -> [w491]
          tunnel: w429 -> [w490]
          tunnel: [w485] -> w425
          tunnel: [w484] -> w424
          tunnel: w423 -> [w483]
          tunnel: [w483] -> w422
          tunnel: w425 -> [w504]
          tunnel: w424 -> [w503]
          tunnel: w422 -> [w501]
          frame #0 {
            n270 = local read "标注图ROI2Mask"() -> (w451:T2)
            n271 = call <vilib>:"Application Directory.vi"() -> ("Application Directory"=w453:path)
            n272 = Concatenate Strings("_" ("字符串"), ".bmp" ("名称或相对路径")) -> (w452:string)
            n273 = Build Path(base path=w453, name or relative path="database\\" ("名称或相对路径")) -> (appended path=w454:path)
            n274 = Build Path(base path=w454, name or relative path=w452) -> (appended path=w444:path)
            "标注后的图片路径" <- w444
            n275 = call <vilib>:"Application Directory.vi"() -> ("Application Directory"=w447:path)
            n276 = call-poly "IMAQ Write File 2"("File Path"=w444, "Image"=w451) -> ()  [unwired: 8 in, 2 out]
            n277 = Build Path(base path=w447, name or relative path="report-template.docx") -> (appended path=w445:path)
          }
          frame #1 {
            n278 = Get Date/Time String(date format (0)=enum16{"short", "long", "abbreviated"}."long" ("日期格式(0)")) -> (date string=w464:string, time string=w465:string)  [unwired: 2 in]
            n279 = call <vilib>:"Create Report.vi"("window state (normal)"=T11."maximized", "report type"=Report_Type."Word", "template (empty)"=w466) -> ("report out"=w461:refnum<class "NI_report.lvclass">, "error out"=w460:errorcluster)  [unwired: 11 in]
            n280 = Concatenate Strings(w464, w465) -> (w459:string)
            n281 = call-poly <vilib>:"Append Report Text.vi"("report in"=w461, "MS Office parameters"=T9 {"position (excel)"={"row"=0, "column"=0}, "name (excel)"="", "bookmark (word)"="time"}, "text"=w459, "error in (no error)"=w460) -> ("report out"=w458:refnum<class "NI_report.lvclass">, "error out"=w457:errorcluster)  [unwired: 8 in, 2 out]
            n282 = call <vilib>:"Word Easy Title.vi"("report in"=w458, "title"="缺陷评定结果", "font"=T10 {"font name"="", "font size"=18.0, "bold"=1, "italic"=0, "underline"=0, "strike through"=0, "font color"=16777216}, "error in (no error)"=w457) -> ("report out"=w472:refnum<class "NI_report.lvclass">, "error out"=w477:errorcluster)  [unwired: 9 in, 1 out]
            n283 = call <vilib>:"Word Easy Text.vi"("report in"=w472, "text"="分层类", "alignment (left)"=enum16{"Left", "Centered", "Right", "Justify"}."Left", "font"=T10 {"font name"="", "font size"=0.0, "bold"=0, "italic"=0, "underline"=0, "strike through"=0, "font color"=16777216}, "error in (no error)"=w477) -> ("report out"=w473:refnum<class "NI_report.lvclass">, "error out"=w474:errorcluster)  [unwired: 8 in, 1 out]
            n284 = call-poly <vilib>:"Word Easy Table.vi"("report in"=w473, "column headers"=string[] ["框号", "长/mm", "宽/mm", "面积/mm2", "Z值", "部位", "类型", "合格性"], "data"=w470, "error in (no error)"=w474) -> ("report out"=w468:refnum<class "NI_report.lvclass">, "error out"=w467:errorcluster)  [unwired: 9 in, 1 out]
          }
          frame #2 {
            n285 = call <vilib>:"Word Easy Text.vi"("report in"=w491, "text"="弥散类", "alignment (left)"=enum16{"Left", "Centered", "Right", "Justify"}."Left", "font"=T10 {"font name"="", "font size"=0.0, "bold"=0, "italic"=0, "underline"=0, "strike through"=0, "font color"=16777216}, "error in (no error)"=w490) -> ("report out"=w494:refnum<class "NI_report.lvclass">, "error out"=w495:errorcluster)  [unwired: 8 in, 1 out]
            n286 = local read "标注后的图片路径"() -> (w486:path)
            n287 = call-poly <vilib>:"Word Easy Table.vi"("report in"=w494, "column headers"=string[] ["框号", "长/mm", "宽/mm", "面积/mm2", "Z值", "部位", "类型", "合格性"], "data"=w492, "error in (no error)"=w495) -> ("report out"=w488:refnum<class "NI_report.lvclass">, "error out"=w487:errorcluster)  [unwired: 9 in, 1 out]
            n288 = call-poly <vilib>:"Append Image to Report.vi"("report in"=w488, "MS Office parameters"=T13 {"position (Excel)"={"row"=0, "column"=0}, "name (Excel)"="", "bookmark (Word)"="image"}, "path or URL of image"=w486, "error in (no error)"=w487) -> ("report out"=w485:refnum<class "NI_report.lvclass">, "error out"=w484:errorcluster)  [unwired: 8 in, 2 out]
          }
          frame #3 {
            n289 = Current VI's Path() -> (path=w506:path)
            n290 = Strip Path(path=w506) -> (stripped path=w510:path)  [unwired: 1 out]
            n291 = Build Path(base path=w510, name or relative path="database\\" ("名称或相对路径")) -> (appended path=w511:path)
            n292 = Concatenate Strings("报表文件.docx" ("名称或相对路径"), w501, ".docx" ("字符串")) -> (w499:string)
            n293 = Build Path(base path=w511, name or relative path=w499) -> (appended path=w507:path)
            n294 = call-dynamic "Save Report to File.vi"("report in"=w504, "report file path"=w507, "error in (no error)"=w503) -> ("report out"=w508:refnum<class "NI_report.lvclass">, "error out"=w509:errorcluster)  [unwired: 11 in]
            n295 = call-dynamic "Dispose Report.vi"("report in"=w508, "error in (no error)"=w509) -> ()  [unwired: 13 in, 1 out]
          }
          frame #4 {
            n296 = One Button Dialog(message="完成评定并退出程序！\n请查看word报告" ("消息")) -> ()  [unwired: 1 in, 1 out]
          }
        }
      }
      event "stop": Value Change {
        # "退出软件"
        n297 = event-data() -> ("NewVal"=w530:bool)  [unwired: 1 in, 4 out]
        n298 = Two Button Dialog(message="是否关闭本软件？" ("消息")) -> (T button?=w532:bool)  [unwired: 2 in]
        n299 = And(x=w530, y=w532) -> (x .and. y?=w529:bool)
        n300 = case shown="真" w529 {
          frame False {
          }
          frame True {
            w533 = TRUE ("All Images? (No)")
            n301 = local read "穿透图"() -> (w535:T2)
            n302 = local read "反射图"() -> (w534:T2)
            n303 = call "IMAQ Dispose"("All Images? (No)"=w533, "Image"=w535) -> ()  [unwired: 4 in, 1 out]
            n304 = call "IMAQ Dispose"("All Images? (No)"=w533, "Image"=w534) -> ()  [unwired: 4 in, 1 out]
            n305 = disable-structure shown="RUN_TIME_ENGINE==True" {
              frame condition #0 {
                n306 = Quit LabVIEW() -> ()  [unwired: 1 in]
              }
              frame condition #1 (active) {
                n307 = Stop() -> ()  [unwired: 1 in]
              }
            }
          }
        }
      }
    }
  }
  "框组" <- T3 [] ("框组")
  "框数" <- 0.0 ("框数")
  "自定义字体" <- T1 {"Desired Font (Application)"=enum."User-specified Font", "[User-specified Font]"={"Font Name"="", "Size"=80, "Strikeout?"=FALSE, "Italic?"=FALSE, "Underline?"=FALSE, "Outline?"=FALSE, "Shadow?"=FALSE, "Bold?"=TRUE, "Rotation Angle"=0.0}, "Horizontal Alignment"=0, "Vertical Alignment"=0} ("Font, Size & Style")
  "部位信息" <- string[] ["", "", "", "", "", "", "", "", ""] ("部位信息")
  "分层类检测结果合并" <- string[][] [] ("弥散类检测结果合并")
  "弥散类检测结果合并" <- string[][] [] ("弥散类检测结果合并")
  "临界Z值" <- 13
  "临界面积百分比值" <- 0.15
